vi "AckNack Response.vi"(8 "error in (no error)":errorcluster, 9 "Original TCP Payload":T2, 10 "Result":T1=enum."RESULT_UNKNOWN", 11 "TCPMessageService in":refnum<class "TCPMessageAPI.lvclass">) -> (0 "error out":errorcluster, 3 "TCPMessageService out":refnum<class "TCPMessageAPI.lvclass">)   [LabVIEW 2020, in "Vecto.lvlib" / "TCPMessageAPI.lvclass"]
uses:
  TCPMessageAPI.lvclass
  proto/TcpPayload/Data.ctl
  proto/AckNackResult/Enumeration.ctl
  proto/TcpAckNack/Data.ctl
  proto/AckNackResult/AckNackResult.lvlib
  proto/TcpAckNack/TcpAckNack.lvlib
  proto/TcpPayload/TcpPayload.lvlib
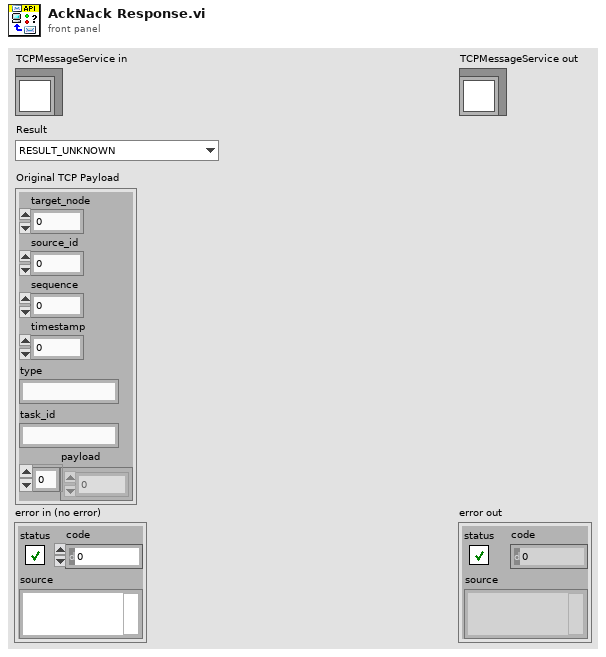
[diagram p1: front panel]
types:
  T1 = typedef "AckNackResult.lvlib/Enumeration.ctl" = enum16{"RESULT_PAYLOAD_ERROR", "RESULT_UNEXPECTED_TYPE", "RESULT_EXPIRED", "RESULT_OUTOFSEQUENCE", "RESULT_DISALLOWED", "RESULT_INVALIDTASK", "RESULT_INVALIDTARGET", "RESULT_UNKNOWN", "RESULT_ACK"}
  T2 = typedef "TcpPayload.lvlib/Data.ctl" = cluster{"target_node":u32, "source_id":u32, "sequence":u32, "timestamp":i64, "type":string, "task_id":string, "payload":u8[]}
  T3 = typedef "TcpAckNack.lvlib/Data.ctl" = cluster{"target_node":u32, "sequence":u32, "timestamp":u64, "type":string, "task_id":string, "result":T1}
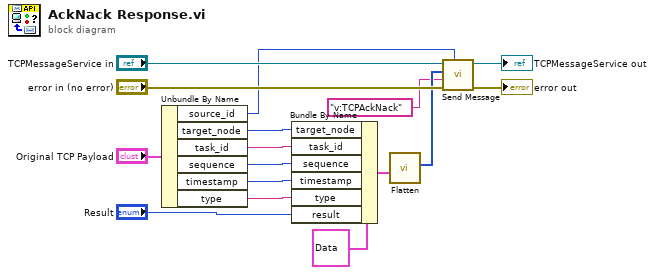
[diagram p0: block diagram]
diagram:
  n1 = Unbundle By Name("Original TCP Payload") -> ("source_id"=w4:u32, "target_node"=w11:u32, "task_id"=w10:string, "sequence"=w9:u32, "timestamp"=w8:i64, "type"=w6:string)
  n2 = Bundle By Name(cluster=T3 {"target_node"=0, "sequence"=0, "timestamp"=0, "type"="", "task_id"="", "result"=enum."RESULT_UNKNOWN"} ("TcpNack"), "target_node"=w11, "task_id"=w10, "sequence"=w9, "timestamp"=w8, "type"=w6, "result"="Result") -> (w7:T3)
  n3 = call "Flatten.vi"("Data"=w7) -> ("Buffer"=w5:u8[])  [unwired: 9 in, 1 out]
  n4 = call "Send Message.vi"("Target ID"=w4, "error in (no error)"="error in (no error)", "Type"="v:TCPAckNack" ("TCPAckNack"), "Payload"=w5, "TCPMessageService in"="TCPMessageService in") -> ("error out"=→"error out":errorcluster, "TCPMessageService out"=→"TCPMessageService out":refnum<class "TCPMessageAPI.lvclass">)  [unwired: 5 in]
